vi "TCP-MultiConn-Server.vi"() -> ()   [LabVIEW 2019]
panel:
  out "#Connections":i32
  out "Chart":dbl(graph)
  in  "SrvPause":bool
  in  "SrvRun":bool
  out "ErrO":errorcluster
  in  "ErrI":errorcluster
  in  "Exit":bool
  # "Server Control"
  # "Run Server to monitor\nthe client connections\nand read and send \ndata to client."
  # "INSTRUCTIONS:\n1. Run Program and server;\n3. Run Client program;\n4. Monitor the data send from Server and received by client."
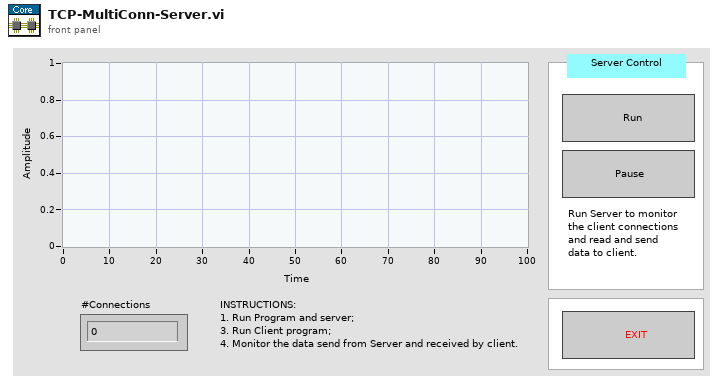
[diagram p1: front panel]
types:
  T1 = cluster{"Clients":refnum<k5>[], "listener ID":refnum<k5>}
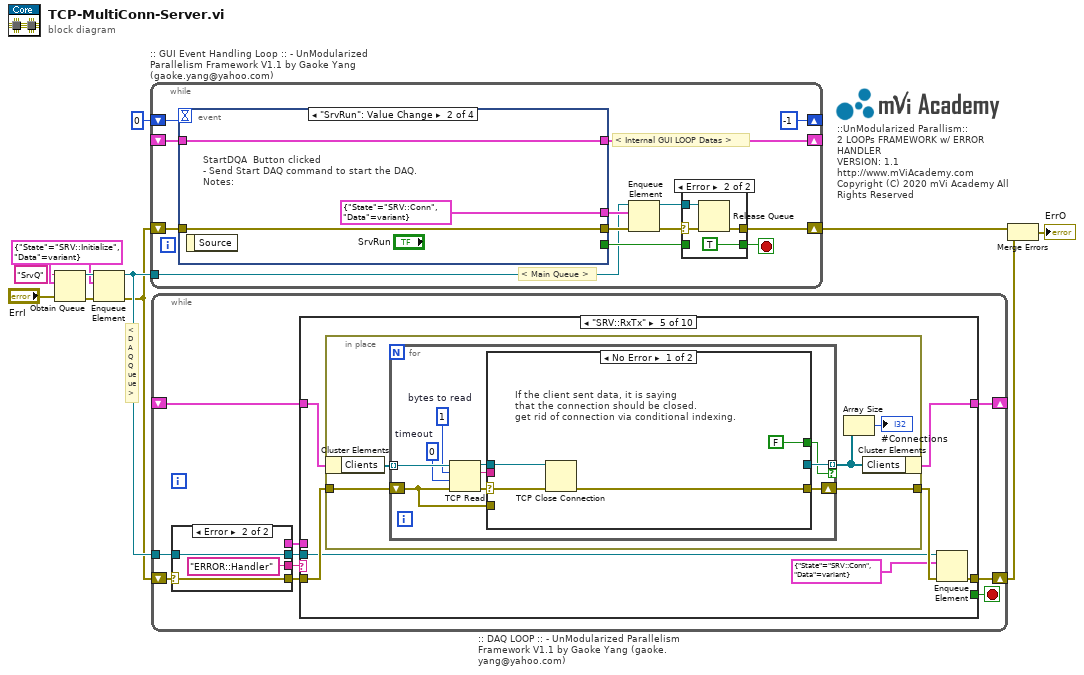
[diagram p0: block diagram]
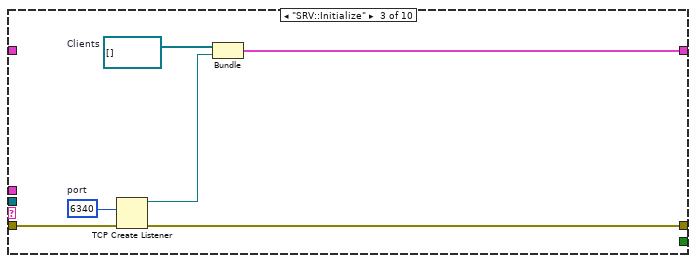
[diagram p4: hidden frame]
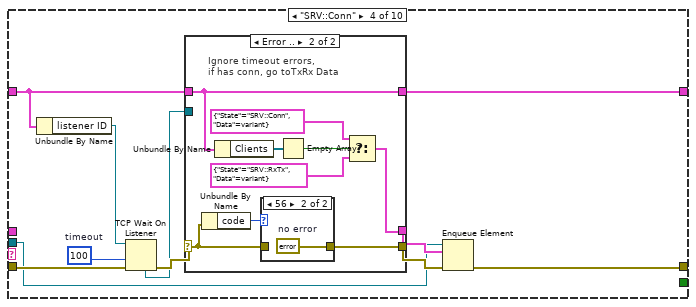
[diagram p5: hidden frame]
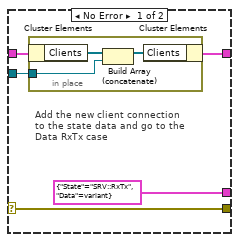
[diagram p6: hidden frame]
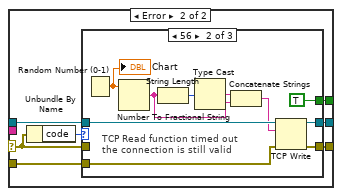
[diagram p8: hidden frame]
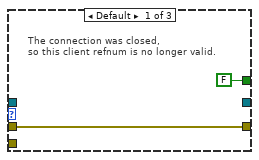
[diagram p9: hidden frame]
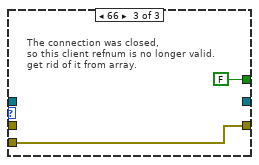
[diagram p10: hidden frame]
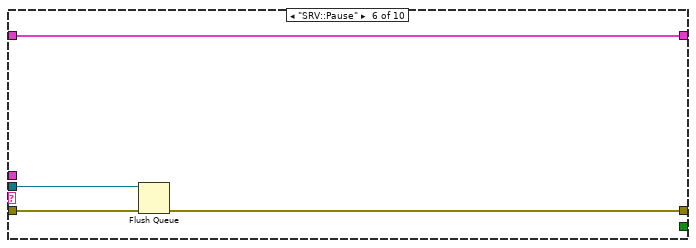
[diagram p11: hidden frame]
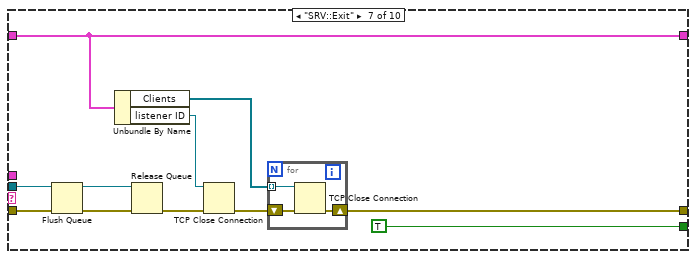
[diagram p12: hidden frame]
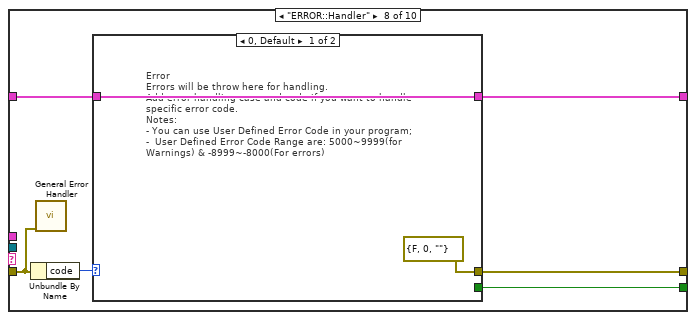
[diagram p13: hidden frame]
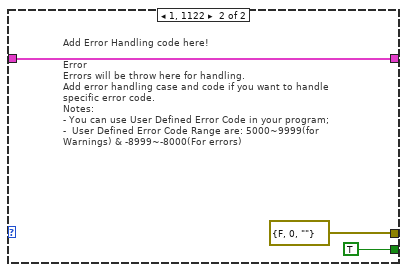
[diagram p14: hidden frame]
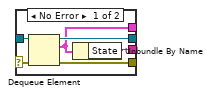
[diagram p17: hidden frame]
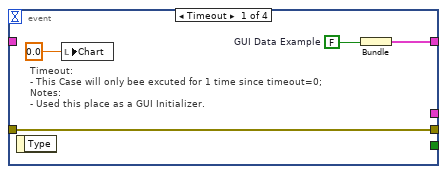
[diagram p19: hidden frame]
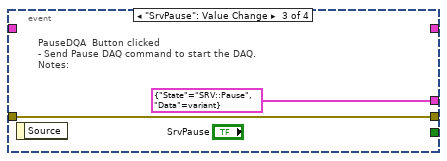
[diagram p20: hidden frame]
diagram:
  w7 = cluster{"State":string, "Data":variant} {"State"="SRV::Initialize", "Data"=variant} ("MainQueue")
  # "::UnModularized Parallism::\n2 LOOPs FRAMEWORK w/ ERROR HANDLER\nVERSION: 1.1\nhttp://www.mViAcademy.com\nCopyright (C) 2020 mVi Academy All Rights Reserved"
  # "< DAQ Queue >"
  n1 = Obtain Queue(name (unnamed)="SrvQ", element data type=w7, error in (no error)="ErrI") -> (queue out=w9:refnum<queue>, error out=w8:errorcluster)  [unwired: 2 in, 1 out]
  n2 = Enqueue Element(queue=w9, element=w7, error in (no error)=w8) -> (queue out=w5:refnum<queue>, error out=w4:errorcluster)  [unwired: 2 out]
  n3 = while ":: GUI Event Handling Loop :: - UnModularized Parallelism Framework V1.1 by Gaoke Yang (gaoke.yang@yahoo.com)" {
    tunnel: w5 -> [w14]
    shift-right: [w23] -> w11
    shift-left: w4 -> [w24]
    shift-right: [-1] -> _
    shift-left: 0 -> [w21]
    shift-right: [w20] -> _
    shift-left: _ -> [w19]
    stop <- w17 stop-if-true
    # "< Internal GUI LOOP Datas >"
    # "< Main Queue >"
    n4 = event shown="[1] \"SrvRun\": Value Change" {
      selector: _ -> [_ _ _ _]
      dyn-events: _ -> [_ _ _ _]
      timeout: w21 -> [_ _ _ _]
      tunnel: [_ _ _ TRUE ("Exit")] -> w18
      tunnel: w24 -> [w34 w37 w39 w40]
      tunnel: [w34 w37 w39 w40] -> w16
      tunnel: [_ cluster{"State":string, "Data":variant} {"State"="SRV::Conn", "Data"=variant} ("MainQueue") cluster{"State":string, "Data":variant} {"State"="SRV::Pause", "Data"=variant} ("MainQueue") cluster{"State":string, "Data":variant} {"State"="SRV::Exit", "Data"=variant} ("Packet")] -> w15
      tunnel: [w32 w36 _ w43] -> w20
      tunnel: w19 -> [_ w36 _ w43]
      event Timeout {
        w33 = FALSE  # GUI Data Example
        # "Timeout:\n- This Case will only bee excuted for 1 time since timeout=0;\nNotes:\n- Used this place as a GUI Initializer."
        n5 = event-data() -> ()  [unwired: 2 out]
        n6 = local write "Chart"(0.0 ("Chart")) -> ()
        n7 = Bundle("GUI Data Example"=w33) -> (w32:cluster{"GUI Data Example":bool})  [unwired: 1 in]
      }
      event "SrvRun": Value Change {
        # "StartDQA  Button clicked\n- Send Start DAQ command to start the DAQ.\nNotes:"
        n8 = event-data() -> ()  [unwired: 2 out]
      }
      event "SrvPause": Value Change {
        # "PauseDQA  Button clicked\n- Send Pause DAQ command to start the DAQ.\nNotes:"
        n9 = event-data() -> ()  [unwired: 2 out]
      }
      event "Exit": Value Change; Panel Close {
        # "Exit Button clicked or panel was closed\n- Send Exit commands and Exit Application\nNotes:"
        n10 = event-data() -> ()  [unwired: 2 out]
      }
    }
    n11 = Enqueue Element(queue=w14, element=w15, error in (no error)=w16) -> (queue out=w12:refnum<queue>, error out=w13:errorcluster)  [unwired: 2 out]
    n12 = case shown="Error" w13 {
      selector: w13 -> [w26 w29]
      tunnel: [w26 w27] -> w23
      tunnel: w18 -> [w25 _]
      tunnel: [w25 TRUE ("Exit")] -> w17
      tunnel: w12 -> [_ w28]
      frame No Error {
      }
      frame Error {
        n13 = Release Queue(queue=w28, error in (no error)=w29) -> (error out=w27:errorcluster)  [unwired: 1 in, 2 out]
      }
    }
  }
  n14 = while ":: DAQ LOOP :: - UnModularized Parallelism Framework V1.1 by Gaoke Yang (gaoke.yang@yahoo.com)" {
    tunnel: w5 -> [w53]
    shift-right: [w47] -> w3
    shift-left: w4 -> [w52]
    shift-right: [w44] -> _
    shift-left: _ -> [w45]
    stop <- w46 stop-if-true
    n15 = case shown="Error" w52 {
      selector: w52 -> [w174 w182]
      tunnel: w53 -> [w179 w180]
      tunnel: [w178 w182] -> w51
      tunnel: [w177 w180] -> w49
      tunnel: [w176 "ERROR::Handler" ("State")] -> w50
      tunnel: [w175 _] -> w48
      frame No Error {
        n16 = Dequeue Element(queue=w179, error in (no error)=w174) -> (queue out=w177:refnum<queue>, element=w175:cluster{"State":string, "Data":variant}, error out=w178:errorcluster)  [unwired: 2 out]
        n17 = Unbundle By Name(w175) -> ("State"=w176:string)
      }
      frame Error {
      }
    }
    n18 = case shown="\"SRV::RxTx\"" w50 {
      tunnel: w51 -> [w54 w57 w58 w67 w100 w142 w154 w160 w171 w173]
      tunnel: [w54 w57 w59 w66 w96 w143 w145 w162 w171 w173] -> w47
      tunnel: [_ _ _ _ _ _ TRUE w161 _ _] -> w46
      tunnel: w49 -> [_ _ _ w65 w95 w141 w153 _ _ _]
      tunnel: [w55 w56 w63 w68 w98 w144 w149 w163 w170 w172] -> w44
      tunnel: w45 -> [w55 w56 _ w64 w99 w144 w149 w164 w170 w172]
      tunnel: w48 -> [_ _ _ _ _ _ _ _ _ _]
      frame "IDLE", Default {
      }
      frame "-------- DAQ ---------" {
      }
      frame "SRV::Initialize" {
        w62 = u16 6340  # port
        w61 = refnum<k5>[] []  # Clients
        n19 = TCP Create Listener(8:w58, 10:w62) -> (0:w59:errorcluster, 3:w60:refnum<k5>)  [unwired: 4 out]
        n20 = Bundle("Clients"=w61, "listener ID"=w60) -> (w63:T1)  [unwired: 1 in]
      }
      frame "SRV::Conn" {
        w72 = 100  # timeout
        n21 = Unbundle By Name(w64) -> ("listener ID"=w70:refnum<k5>)
        n22 = TCP Wait On Listener(8:w67, 9:w72, 11:w70) -> (0:w71:errorcluster, 4:w69:refnum<k5>)  [unwired: 4 out]
        n23 = case shown="Error .." w71 {
          selector: w71 -> [w79 w91]
          tunnel: [w79 w89] -> w73
          tunnel: w69 -> [w78 _]
          tunnel: w64 -> [w77 w86]
          tunnel: [w76 w86] -> w68
          tunnel: [cluster{"State":string, "Data":variant} {"State"="SRV::RxTx", "Data"=variant} ("MainQueue") w83] -> w74
          frame No Error {
            # "Add the new client connection \nto the state data and go to the \nData RxTx case"
            n24 = in-place {
              in-place-border: w78 -> [w80]
              n25 = in-place-cluster #1(w77) -> ("Clients"=w82:refnum<k5>[])
              n26 = Build Array (concatenate)(w82, w80) -> (w81:refnum<k5>[])
              n27 = in-place-cluster #1("Clients"=w81) -> (w76:T1)
            }
          }
          frame Error {
            # "Ignore timeout errors, \nif has conn, go toTxRx Data"
            n28 = Unbundle By Name(w91) -> ("code"=w90:i32)
            n29 = Unbundle By Name(w86) -> ("Clients"=w88:refnum<k5>[])
            n30 = case shown="56" w90 {
              tunnel: w91 -> [w92 _]
              tunnel: [w92 w93] -> w89
              frame Default {
              }
              frame 56 {
                w93 = errorcluster {"status"=FALSE, "code"=0, "source"=""}  # no error
              }
            }
            n31 = Empty Array?(array=w88) -> (empty?=w87:bool)
            n32 = Select(t=cluster{"State":string, "Data":variant} {"State"="SRV::Conn", "Data"=variant} ("MainQueue"), s=w87, f=cluster{"State":string, "Data":variant} {"State"="SRV::RxTx", "Data"=variant} ("MainQueue")) -> (s? t:f=w83:cluster{"State":string, "Data":variant})
          }
        }
        n33 = Enqueue Element(queue=w65, element=w74, error in (no error)=w73) -> (error out=w66:errorcluster)  [unwired: 3 out]
      }
      frame "SRV::RxTx" {
        n34 = in-place {
          in-place-border: w100 -> [w104]
          in-place-border: [w103] -> w97
          n35 = in-place-cluster #2(w99) -> ("Clients"=w105:refnum<k5>[])
          n36 = for {
            tunnel: w105 -> [w115] mode=indexing
            shift-right: [w111] -> w103
            shift-left: w104 -> [w106]
            tunnel: [w108] -> w101 mode=indexing if=w107
            w109 = 0  # timeout
            w110 = 1  # bytes to read
            n37 = TCP Read(connection ID=w115, bytes to read=w110, error in (no error)=w106, 9:w109) -> (connection ID out=w112:refnum<k5>, data out=w113:string, error out=w114:errorcluster)  [unwired: 1 out]
            n38 = case shown="No Error" w114 {
              selector: w114 -> [w119 w124]
              tunnel: w113 -> [_ _]
              tunnel: w112 -> [w118 w123]
              tunnel: [w117 w125] -> w111
              tunnel: [_ w122] -> w108
              tunnel: [FALSE w121] -> w107
              tunnel: w106 -> [_ w120]
              frame No Error {
                # "If the client sent data, it is saying \nthat the connection should be closed.\nget rid of connection via conditional indexing."
                n39 = TCP Close Connection(connection ID=w118, error in (no error)=w119) -> (error out=w117:errorcluster)  [unwired: 2 out]
              }
              frame Error {
                n40 = Unbundle By Name(w124) -> ("code"=w126:i32)
                n41 = case shown="56" w126 {
                  tunnel: [w127 w135 w139] -> w125
                  tunnel: w124 -> [w127 _ _]
                  tunnel: w123 -> [_ w134 _]
                  tunnel: [_ w133 _] -> w122
                  tunnel: [FALSE TRUE FALSE] -> w121
                  tunnel: w120 -> [_ w129 w139]
                  frame Default {
                    # "The connection was closed, \nso this client refnum is no longer valid."
                  }
                  frame 56 {
                    # "TCP Read function timed out\nthe connection is still valid"
                    n42 = Random Number (0-1)() -> (number: 0 to 1=w130:dbl)
                    "Chart" <- w130
                    n43 = Number To Fractional String(number=w130) -> (F-format string=w136:string)  [unwired: 3 in]
                    n44 = String Length(string=w136) -> (length=w137:i32)
                    n45 = Type Cast(x=w137) -> (*(type *) &x=w138:string)  [unwired: 1 in]
                    n46 = Concatenate Strings(w138, w136) -> (w132:string)
                    n47 = TCP Write(connection ID=w134, data in=w132, error in (no error)=w129) -> (connection ID out=w133:refnum<k5>, error out=w135:errorcluster)  [unwired: 2 out]
                  }
                  frame 66 {
                    # "The connection was closed, \nso this client refnum is no longer valid.\nget rid of it from array."
                  }
                }
              }
            }
          }
          n48 = Array Size(array=w101) -> (size(s)=→"#Connections":i32)
          n49 = in-place-cluster #2("Clients"=w101) -> (w98:T1)
        }
        n50 = Enqueue Element(queue=w95, element=cluster{"State":string, "Data":variant} {"State"="SRV::Conn", "Data"=variant} ("MainQueue"), error in (no error)=w97) -> (error out=w96:errorcluster)  [unwired: 3 out]
      }
      frame "SRV::Pause" {
        n51 = Flush Queue(queue=w141, error in (no error)=w142) -> (error out=w143:errorcluster)  [unwired: 2 out]
      }
      frame "SRV::Exit" {
        n52 = Flush Queue(queue=w153, error in (no error)=w154) -> (queue out=w151:refnum<queue>, error out=w152:errorcluster)  [unwired: 1 out]
        n53 = Unbundle By Name(w149) -> ("Clients"=w147:refnum<k5>[], "listener ID"=w148:refnum<k5>)
        n54 = Release Queue(queue=w151, error in (no error)=w152) -> (error out=w146:errorcluster)  [unwired: 1 in, 2 out]
        n55 = TCP Close Connection(connection ID=w148, error in (no error)=w146) -> (error out=w150:errorcluster)  [unwired: 1 in, 1 out]
        n56 = for {
          shift-right: [w157] -> w145
          shift-left: w150 -> [w158]
          tunnel: w147 -> [w156] mode=indexing
          n57 = TCP Close Connection(connection ID=w156, error in (no error)=w158) -> (error out=w157:errorcluster)  [unwired: 1 in, 1 out]
        }
      }
      frame "ERROR::Handler" {
        n58 = Unbundle By Name(w160) -> ("code"=w159:i32)
        n59 = call <vilib>:"General Error Handler.vi"("error in (no error)"=w160) -> ()  [unwired: 10 in, 5 out]
        n60 = case shown="0, Default" w159 {
          tunnel: [w166 w169] -> w163
          tunnel: w164 -> [w166 w169]
          tunnel: [errorcluster {"status"=FALSE, "code"=0, "source"=""} ("error out") errorcluster {"status"=FALSE, "code"=0, "source"=""} ("error out")] -> w162
          tunnel: [_ TRUE] -> w161
          frame 0, Default {
            # "Error\nErrors will be throw here for handling.\nAdd error handling case and code if you want to handle specific error code.\nNotes:\n- You can use User Defined Error Code in your program;\n-  User Defined Error Code Range are: 5000~9999(for Warnings) & -8999~-8000(For errors)"
          }
          frame 1, 1122 {
            # "Add Error Handling code here!\n\nError\nErrors will be throw here for handling.\nAdd error handling case and code if you want to handle specific error code.\nNotes:\n- You can use User Defined Error Code in your program;\n-  User Defined Error Code Range are: 5000~9999(for Warnings) & -8999~-8000(For errors)"
          }
        }
      }
      frame "--------User Case---------" {
      }
      frame "Reserved" {
      }
    }
  }
  n61 = Merge Errors(w11, w3) -> (→"ErrO":errorcluster)
